vi "Time Stamp or Now.vi"(1 "time stamp in":timestamp) -> (0 "time stamp out":timestamp)   [LabVIEW 2020, in "PV Access.lvlib" / "PV Data.lvlib"]
uses:
  PV Data.lvlib
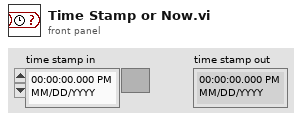
[diagram p1: front panel]
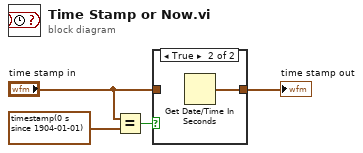
[diagram p0: block diagram]
diagram:
  n1 = Equal?(x="time stamp in", y=timestamp(0 s since 1904-01-01) ("timestamp 2")) -> (x = y?=w4:bool)
  n2 = case shown="True" w4 {
    tunnel: "time stamp in" -> [w5 _]
    tunnel: [w5 w6] -> w1
    frame False {
    }
    frame True {
      n3 = Get Date/Time In Seconds() -> (seconds since 1Jan1904=w6:timestamp)
    }
  }
  "time stamp out" <- w1
